vi "Belkin Demo Image Proc V2.vi"() -> ()   [LabVIEW 2015]
uses:
  <vilib>/userdefined/High Color/IMAQdx.ctl
  <vilib>/Platform/TimedLoop/XDataNode/timing_clust.ctl
  <vilib>/Platform/TimedLoop/XDataNode/nitl_modes.ctl
  <vilib>/Platform/TimedLoop/XDataNode/wakeup.ctl
  <vilib>/FPGAPlugInAG/cRIO-9030/niLvFpga_Open_cRIO-9030.vi
  <vilib>/rvi/interface/common/dynamic/niFpgaDynamicAddResources.vi
  <vilib>/FPGAPlugInAG/Dynamic/niLvFpga_Abort_Dynamic.vi
  <vilib>/FPGAPlugInAG/Dynamic/niLvFpga_Run_Dynamic.vi
  <vilib>/Utility/error.llb/Error Cluster From Error Code.vi
  <vilib>/rvi/errors/niLvFpgaAdjustHostInterfaceError.vi
  <vilib>/FPGAPlugInAG/Dynamic/niLvFpga_Close_Dynamic.vi
  <vilib>/rvi/interface/nirviOpenFPGA/nirviOpenFPGA.xnode
  FPGA Bitfiles/BelkinDemo_FPGATarget_BelkinPolartoCom_2zVnbe-nqac.lvbitx
  FPGA/Belkin Polar to Complex.vi
  <vilib>/rvi/interface/nirviMethod/nirviMethod.xnode
  <vilib>/rvi/interface/nirviReadWriteControl/nirviReadWriteControl.xnode
  <vilib>/rvi/interface/nirviCloseFPGA/nirviCloseFPGA.xnode
  <vilib>/Platform/TimedLoop/XDataNode/XDataNode.xnode
  <vilib>/vision/driver/NI_Vision_Acquisition_Software.lvlib
  NiFpgaLv.dll
  <vilib>/rvi/interface/Simulation/niFpgaSimulationCallBeginRW.vi
  <vilib>/Platform/TimedLoop/XDataNode/XDNodeRunTimeDep.lvlib
panel:
  in  "DesiredRange":u32=508206
  in  "AutoRange":bool=TRUE
  out "MaximalHist":sgl=507915.0
  in  "DesiredHist":i32=40
  in  "ExpGain":i32=-100
  in  "AutoExposure":bool=TRUE
  out "HistMax":i32=38
  in  "Source":bool=TRUE
  in  "Exposure":u32=85000
  in  "Pause":bool
  in  "File Path":path=path "/home/lvuser/Images/yuval eye 6.png"
  in  "Radius Delta":dbl
  in  "Auto Radius":bool=TRUE
  in  "Debug Overlay":bool
  in  "Y Overlay":sgl=452.0
  in  "X Overlay":sgl=620.0
  out "Image Proc Error":errorcluster
  in  "ScanContinues":bool=TRUE
  out "Center (Pixels)":cluster{"X":sgl, "Y":sgl}
  in  "Decimator":u16=65535
  in  "EngleDelta":fxp<+/-,16,1>=0.06005859375
  in  "EndEngle":fxp<+/-,16,2>=1.99993896484375
  in  "StartAngle":fxp<+,16,2>
  in  "Radius (Pixels)":dbl=281.0
  in  "Yofset":fxp<+/-,16,16>=493.0
  in  "Xofset":fxp<+/-,16,16>=470.0
  in  "Ygain":fxp<+/-,32,1>=0.001459998544305563
  in  "Xgain":fxp<+/-,32,1>=-0.001459999941289425
  in  "Y Scanner":sgl=512.0
  in  "X Scanner":sgl=640.0
  in  "Debug Scanner Center":bool
  out "Cycle":u32=162
  in  "Threshold":cluster{"Lower value":sgl, "Upper value":sgl}={"Lower value"=0.0, "Upper value"=150.0}
  out "Fitted Circle":T1
  out "FPGA Ref Error":errorcluster
  out "Image Acq. Error":errorcluster
  in  "Session In":T2="cam0"
  out "Image Out":T3(plugin-control)
  in  "stop":bool=TRUE
  # "Image Poc. Params"
  # "Calibration Params"
  # "Scan Params"
  # "Scan Speed Params"
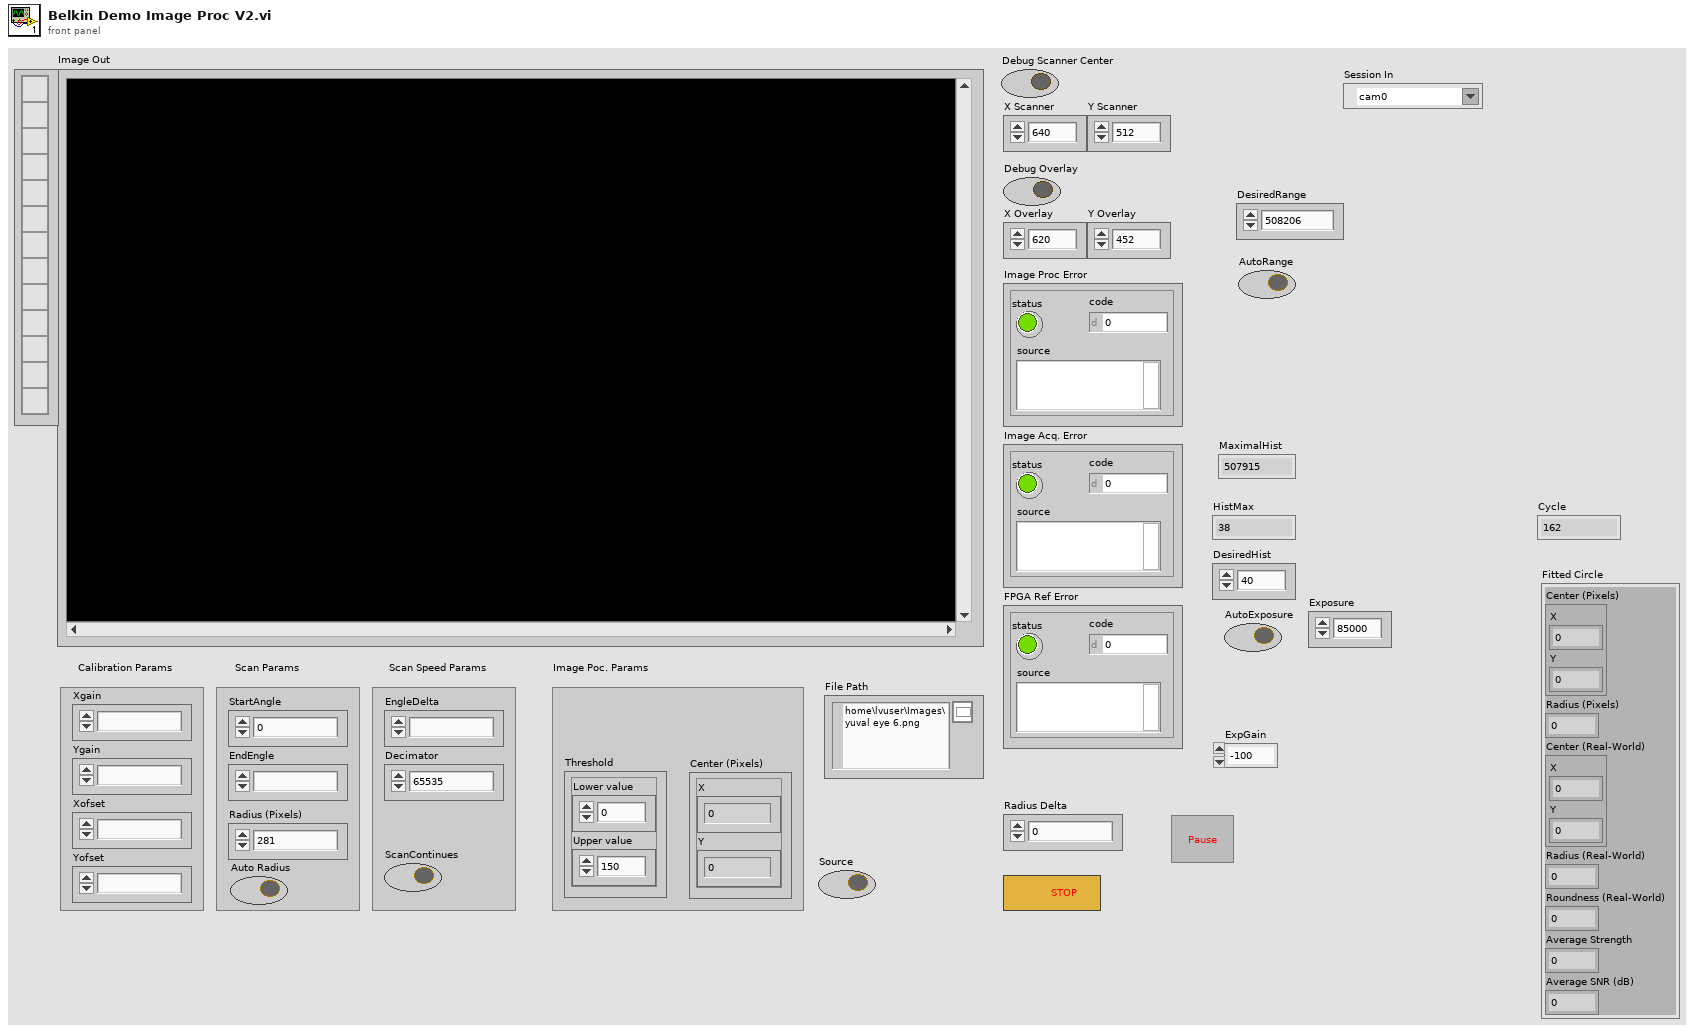
[diagram p1: front panel]
types:
  T1 = cluster{"Center (Pixels)":cluster{"X":sgl, "Y":sgl}, "Radius (Pixels)":dbl, "Center (Real-World)":cluster{"X":sgl, "Y":sgl}, "Radius (Real-World)":dbl, "Roundness (Real-World)":dbl, "Average Strength":dbl, "Average SNR (dB)":dbl}
  T2 = typedef "IMAQdx.ctl" = refnum<k21>
  T3 = typedef "IMAQ Image.ctl" = refnum<image>
  T4 = typedef "Image Type" = u32
  T5 = typedef "XDNodeRunTimeDep.lvlib/timing_clust.ctl" = cluster{"Expected End [f-1]":u64, "Actual End [f-1]":u64, "Finished Late? [f-1]":bool, "Expected End [i-1]":u64, "Actual End [i-1]":u64, "Finished Late? [i-1]":bool, "Expected Start [i]":u64, "Actual Start [i]":u64, "Expected Start [f]":u64, "Actual Start [f]":u64, "Source Name":string, "Structure Name":string, "Period":i64, "Deadline":i64, "Offset":i64, "Start":i64, "Priority":i32, "Timeout":i32, "Mode":T6, "Wakeup Reason":T7, "Error":errorcluster, "Source Type":string, "Secondary Source Type":string, "Global End Time":u64, "Global Start Time":u64, "Frame Duration":u64, "Iteration Duration":u64, "Assigned CPU":i32, "I/O Scan Engine Mode":u32}
  T6 = typedef "XDNodeRunTimeDep.lvlib/nitl_modes.ctl" = enum32{"No Change", "Process missed periods, maintain original phase", "Discard missed periods, maintain original phase", "Process missed periods, ignore original phase", "Discard missed periods, ignore original phase"}
  T7 = typedef "XDNodeRunTimeDep.lvlib/wakeup.ctl" = enum32{"Normal", "Aborted", "Asynchronous wakeup", "Timing source error", "Timed loop error", "Timeout"}
  T8 = cluster{"Position":cluster{"X":sgl, "Y":sgl}, "Radius":dbl, "Score":dbl}
  T9 = cluster{"Position":cluster{"X":sgl, "Y":sgl}, "Radius":dbl, "Score":dbl}[]
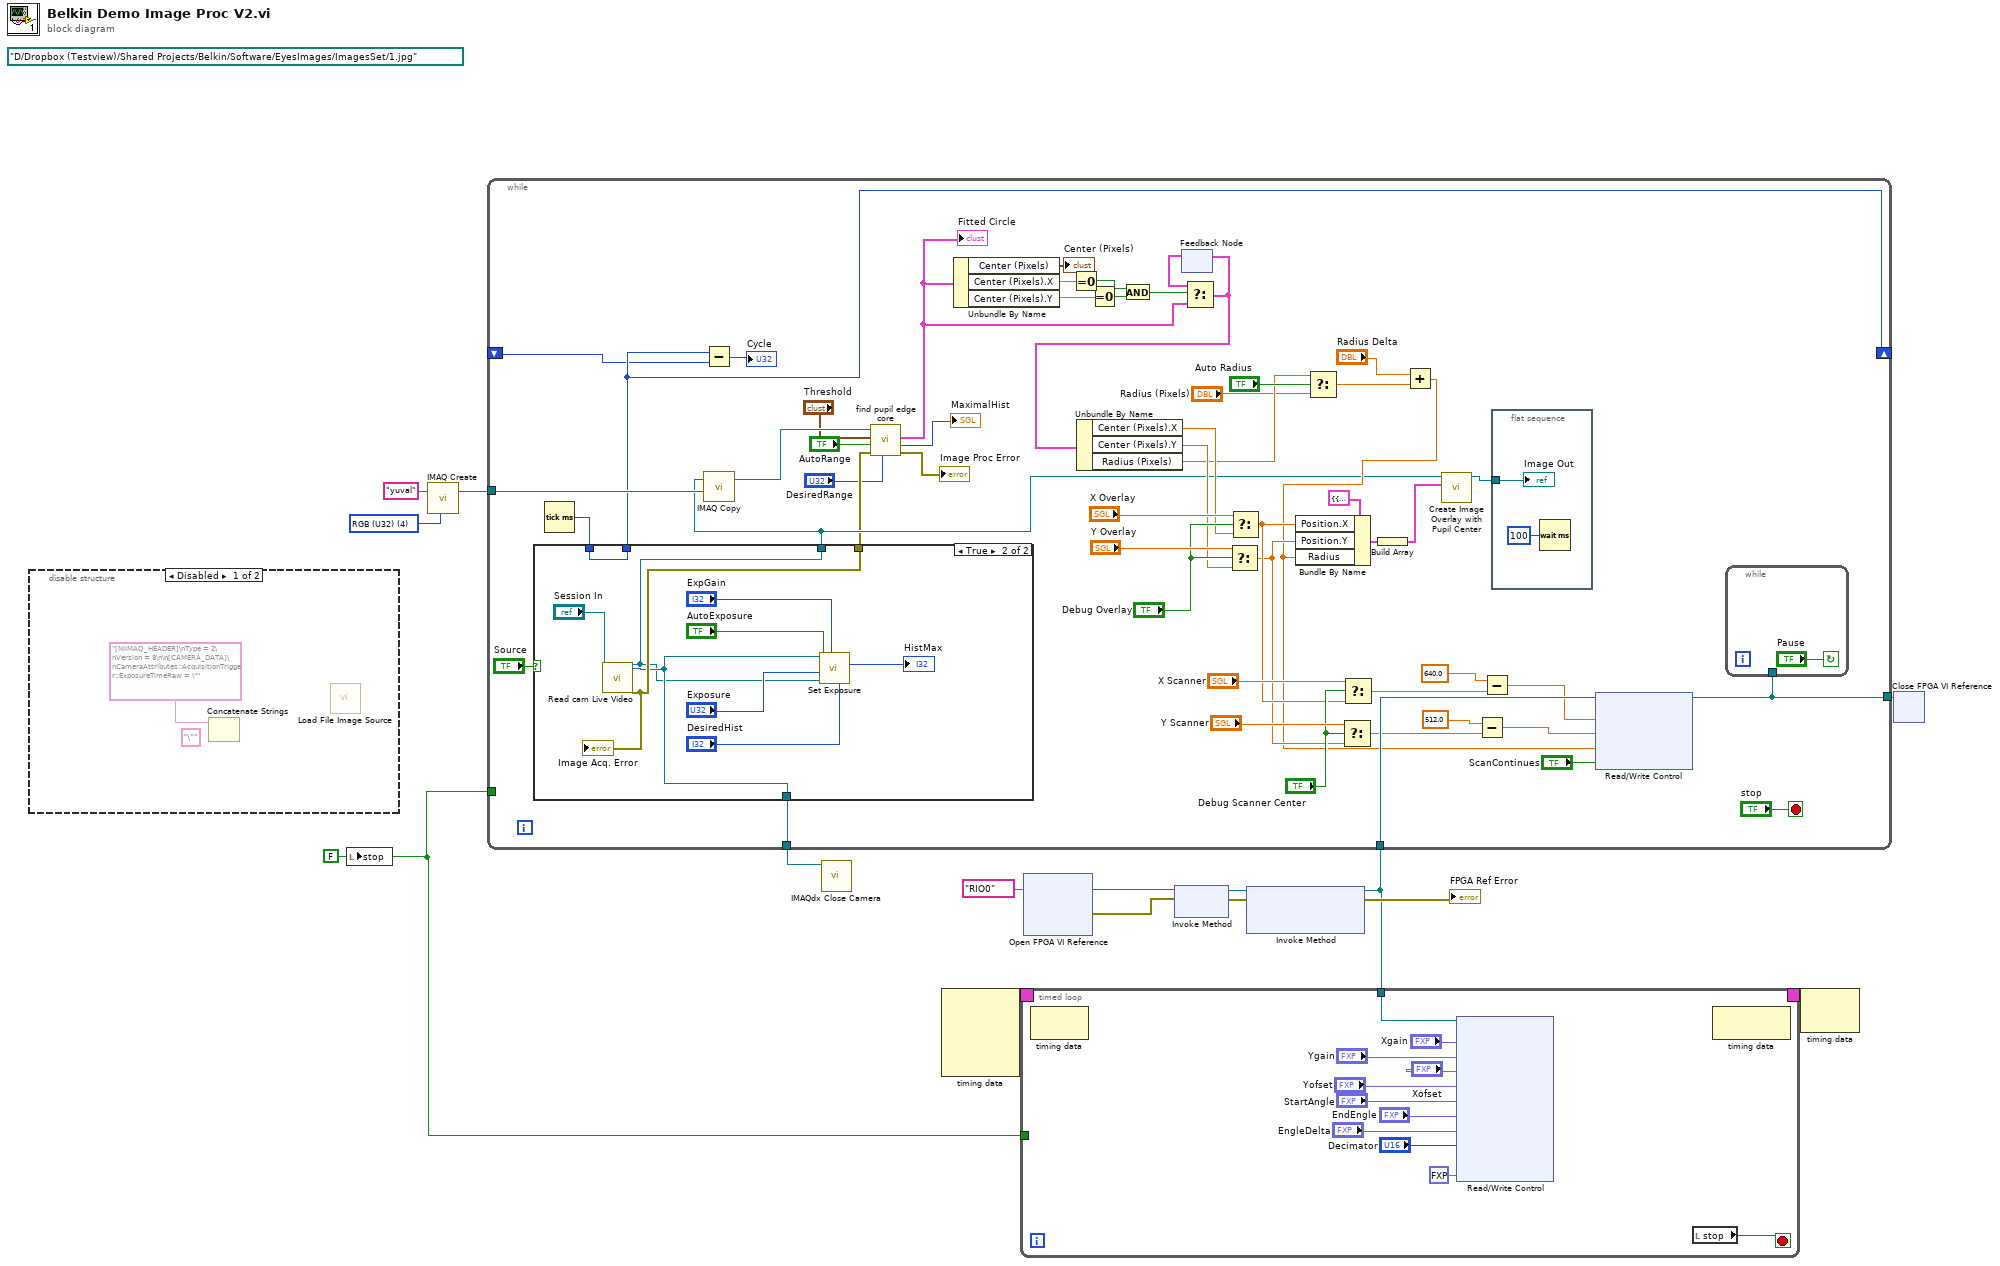
[diagram p0: block diagram]
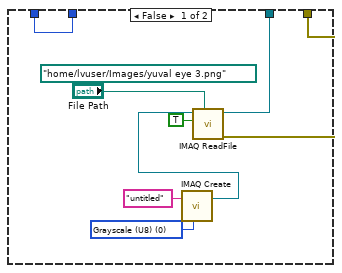
[diagram p2: hidden frame]
diagram:
  w1 = FALSE ("stop")
  w14 = T4 4 items=["Grayscale (U8)", "Grayscale (I16)", "Grayscale (SGL)", "Complex (CSG)", "RGB (U32)", "HSL (U32)", "RGB (U64)", "Grayscale (U16)"] ("Image Type")
  (unwired) path "D:/Dropbox (Testview)/Shared Projects/Belkin/Software/EyesImages/ImagesSet/1.jpg" ("File Path")
  n1 = disable-structure shown="Disabled" {
    frame Disabled {
      (unwired) "\"" ("string")
      n2 = Concatenate Strings("[NIIMAQ_HEADER]\nType = 2\nVersion = 8\n\n[CAMERA_DATA]\nCameraAttributes::AcquisitionTrigger::ExposureTimeRaw = \"") -> (w17:string)  [unwired: 1 in, 1 out]
      n3 = call "Load File Image Source.vi"() -> ()  [unwired: 10 in, 2 out]
    }
    frame Enabled {
    }
  }
  n4 = local write "stop"(w1) -> ()
  n5 = call "IMAQ Create"("Image Name"="yuval", "Image Type"=w14) -> ("New Image"=w12:T3)  [unwired: 2 in, 2 out]
  n6 = node-c288() -> (w3:T5)  [unwired: 4 in]
  n7 = xnode "Open FPGA VI Reference"("resource name"=tag "RIO0") -> ("FPGA VI Reference Out"=w7:refnum<k20>, "error out"=w5:errorcluster)  [unwired: 1 in]
  n8 = xnode "Invoke Method"("FPGA VI Reference In"=w7, "error in"=w5) -> ("FPGA VI Reference Out"=w9:refnum<k20>, "error out"=w8:errorcluster)
  n9 = xnode "Invoke Method"("FPGA VI Reference In"=w9, "error in"=w8) -> ("FPGA VI Reference Out"=w4:refnum<k20>, "error out"=→"FPGA Ref Error":errorcluster)  [unwired: 1 in]
  n10 = while {
    tunnel: [w70] -> w15
    tunnel: w12 -> [w69]
    tunnel: w4 -> [w68]
    tunnel: [w25] -> w10
    shift-right: [w62] -> _
    shift-left: _ -> [w61]
    tunnel: w1 -> [_]
    stop <- "stop" stop-if-true
    n11 = Tick Count (ms)() -> (millisecond timer value=w22:u32)
    n12 = case shown="True" "Source" {
      tunnel: [_ w82] -> w70
      tunnel: [w72 w89] -> w62
      tunnel: [w74 w80] -> w24
      tunnel: [w73 w87] -> w23
      tunnel: w22 -> [w72 w89]
      frame False {
        w76 = T4 0 items=["Grayscale (U8)", "Grayscale (I16)", "Grayscale (SGL)", "Complex (CSG)", "RGB (U32)", "HSL (U32)", "RGB (U64)", "Grayscale (U16)"] ("Image Type")
        (unwired) path "/home/lvuser/Images/yuval eye 3.png" ("File Path")
        n13 = call "IMAQ Create"("Image Name"="untitled", "Image Type"=w76) -> ("New Image"=w77:T3)  [unwired: 2 in, 2 out]
        n14 = call "IMAQ ReadFile"("File Path"="File Path", "Load Color Palette? (No)"=TRUE, "Image"=w77) -> ("error out"=w73:errorcluster, "Image Out"=w74:T3)  [unwired: 4 in, 3 out]
      }
      frame True {
        n15 = call "Read cam Live Video.vi"("Session In"="Session In") -> ("Image Out"=w80:T3, "Session Out"=w82:T2, "error out"=w87:errorcluster)  [unwired: 24 in]
        "Image Acq. Error" <- w87
        n16 = call "Set Exposure.vi"("DesiredHist"="DesiredHist", "ExpGain"="ExpGain", "Image"=w80, "Exposure"="Exposure", "AutoExposure"="AutoExposure", "Session Out"=w82) -> ("HistMax"=→"HistMax":i32)  [unwired: 5 in]
      }
    }
    n17 = Subtract(x=w62, y=w61) -> (x-y=→"Cycle":u32)
    n18 = call "IMAQ Copy"("Image Dst"=w69, "Image Src"=w24) -> ("Image Dst Out"=w67:T3)  [unwired: 1 in, 4 out]
    n19 = call "find pupil edge core.vi"("DesiredRange"="DesiredRange", "error in (no error)"=w23, "AutoRange"="AutoRange", "Range"="Threshold", "Refnum in"=w67) -> ("error out"=→"Image Proc Error":errorcluster, "MaxHist"=→"MaximalHist":i32, "Fitted Circle"=w34:T1)  [unwired: 3 in, 1 out]
    "Fitted Circle" <- w34
    n20 = Unbundle By Name(w34) -> ("Center (Pixels)"=→"Center (Pixels)":cluster{"X":sgl, "Y":sgl}, "Center (Pixels).X"=w39:sgl, "Center (Pixels).Y"=w38:sgl)
    n21 = Equal To 0?(x=w39) -> (x = 0?=w36:bool)
    n22 = Equal To 0?(x=w38) -> (x = 0?=w37:bool)
    n23 = And(x=w36, y=w37) -> (x .and. y?=w35:bool)
    n24 = feedback #1() -> (w32:T1)  [unwired: 1 in]
    n25 = Select(t=w32, s=w35, f=w34) -> (s? t:f=w33:T1)
    n26 = Unbundle By Name(w33) -> ("Center (Pixels).X"=w42:sgl, "Center (Pixels).Y"=w41:sgl, "Radius (Pixels)"=w30:dbl)
    n27 = feedback-in #1(w33) -> ()
    n28 = Select(t="Y Overlay", s="Debug Overlay", f=w41) -> (s? t:f=w44:sgl)
    n29 = Select(t="X Overlay", s="Debug Overlay", f=w42) -> (s? t:f=w45:sgl)
    n30 = Select(t=w30, s="Auto Radius", f="Radius (Pixels)") -> (s? t:f=w27:dbl)
    n31 = Select(t="Y Scanner", s="Debug Scanner Center", f=w44) -> (s? t:f=w52:sgl)
    n32 = Select(t="X Scanner", s="Debug Scanner Center", f=w45) -> (s? t:f=w53:sgl)
    n33 = Add(x="Radius Delta", y=w27) -> (x+y=w26:dbl)
    n34 = Bundle By Name(cluster=T8 {"Position"={"X"=0.0, "Y"=0.0}, "Radius"=0.0, "Score"=0.0} ("Circle Descriptor"), "Position.X"=w45, "Position.Y"=w44, "Radius"=w26) -> (w56:T8)
    n35 = Build Array(w56) -> (w55:T9)
    n36 = call "Create Image Overlay with Pupil Center.vi"("Circles"=w55, "Refnum in"=w24) -> ("Refnum out"=w58:T3)  [unwired: 9 in]
    n37 = Subtract(x=512.0, y=w52) -> (x-y=w63:dbl)
    n38 = Subtract(x=640.0, y=w53) -> (x-y=w65:dbl)
    n39 = flat-sequence {
      tunnel: w58 -> [w92]
      frame #0 {
        n40 = Wait (ms)(milliseconds to wait=u32 100) -> ()  [unwired: 1 out]
        "Image Out" <- w92
      }
    }
    n41 = xnode "Read/Write Control"("FPGA VI Reference In"=w68, "Xpos"=w65, "Ypos"=w63, "PupilRadius"=w26, "ScanContinues"="ScanContinues") -> ("FPGA VI Reference Out"=w25:refnum<k20>)  [unwired: 1 in, 1 out]
    n42 = while {
      tunnel: w25 -> [_]
      stop <- "Pause" continue-if-true
    }
  }
  n43 = call <vilib>:"IMAQdx Close Camera.vi"("Session In"=w15) -> ()  [unwired: 1 in, 10 out]
  n44 = timed-loop {
    tunnel: w4 -> [w103]
    timing: w3 -> [_]
    timing-out: [_] -> w2
    tunnel: w1 -> [_]
    stop <- w93 stop-if-true
    w98 = fxp<+/-,20,5> 5.0 ("Max_X_Voltage")
    n45 = node-c288() -> ()  [unwired: 1 in, 1 out]
    n46 = xnode "Read/Write Control"("FPGA VI Reference In"=w103, "Xgain"="Xgain", "Ygain"="Ygain", "Xofset"="Xofset", "Yofset"="Yofset", "StartAngle"="StartAngle", "EndEngle"="EndEngle", "EngleDelta"="EngleDelta", "Decimator"="Decimator", "Max_X_Voltage"=w98, "Max_Y_Voltage"=w98) -> ()  [unwired: 1 in, 2 out]
    n47 = local read "stop"() -> (w93:bool)
    n48 = node-c288() -> ()  [unwired: 1 in, 1 out]
  }
  n49 = node-c288(w2) -> ()  [unwired: 1 out]
  n50 = xnode "Close FPGA VI Reference"("FPGA VI Reference In"=w10) -> ()  [unwired: 1 in, 1 out]
